vi "Global.vi"() -> ()   [LabVIEW 2020]
panel:
  in  "校验码":string
  in  "图号":string
  in  "法规号":string
  out "设备状态":i32
  in  "软件版本号":string
  in  "白/夜班":string
  in  "返工码":string
  in  "追溯代码":string
  in  "操作步骤":bool[](array[boolean])
  in  "更换型号":refnum<vi>
  in  "产品引用":refnum<vi>
  out "扭矩 2":sgl format="%#.3f"
  in  "扭矩":refnum<vi>
  out "传感器读数":T1 {"吸收电流" format="%#.3f"; "输出扭矩(大)" format="%#.3f"; "输出扭矩(小)" format="%#.3f"; "输入扭矩" format="%#.3f"; "输入编码位移" format="%#.3f"; "工装移载位移" format="%#.3f"; "输入移载位移" format="%#.3f"; "扭矩" format="%#.3f"}
  in  "CRC计数":u8
  in  "CAN_CYCLE":T2(array[cluster]) {"周期(ms)" min=1 format="%d ms"; "ID" format="0x%x"}
  in  "STOP_CAN":bool
  out "当前车速":u16
  in  "CAN Info":T3={"波特率"=11, "ID"=0, "帧类型"=enum."标准帧", "帧格式"=enum."数据帧", "周期(ms)"=10} {"周期(ms)" min=1 format="%d ms"; "ID" format="0x%x"; "波特率" items=["5Kbps", "10Kbps", "20Kbps", "40Kbps", "50Kbps", "80Kbps", "100Kbps", "125Kbps", "200Kbps", "250Kbps", "400Kbps", "500Kbps", "666Kbps", "800Kbps", "1000Kbps"]}
  in  "启用CAN":bool
  in  "合格数量 2":i32
  in  "生产数量 2":i32
  in  "计时开始":bool
  in  "计时复位":bool
  in  "前序状态":refnum<vi>
  in  "前序显示字":refnum<vi>
  in  "产品型号":string(combo)
  in  "结果显示":refnum<vi>
  in  "result":string
  in  "检测结果":refnum<vi>
  in  "合格数量":refnum<vi>
  in  "生产数量":refnum<vi>
  out "模式":u32
  in  "更换产品":refnum<vi>
  in  "提示信息":refnum<vi>
  in  "程序自动":refnum<vi>
  in  "报警图标":refnum<vi>
  in  "程序关闭":bool
  in  "Info":refnum<vi>
  in  "Result":refnum<vi>
  in  "批次":refnum<vi>
  # "帧ID"
  # "帧类型"
  # "帧格式"
  # "帧数据"
  # "周期"
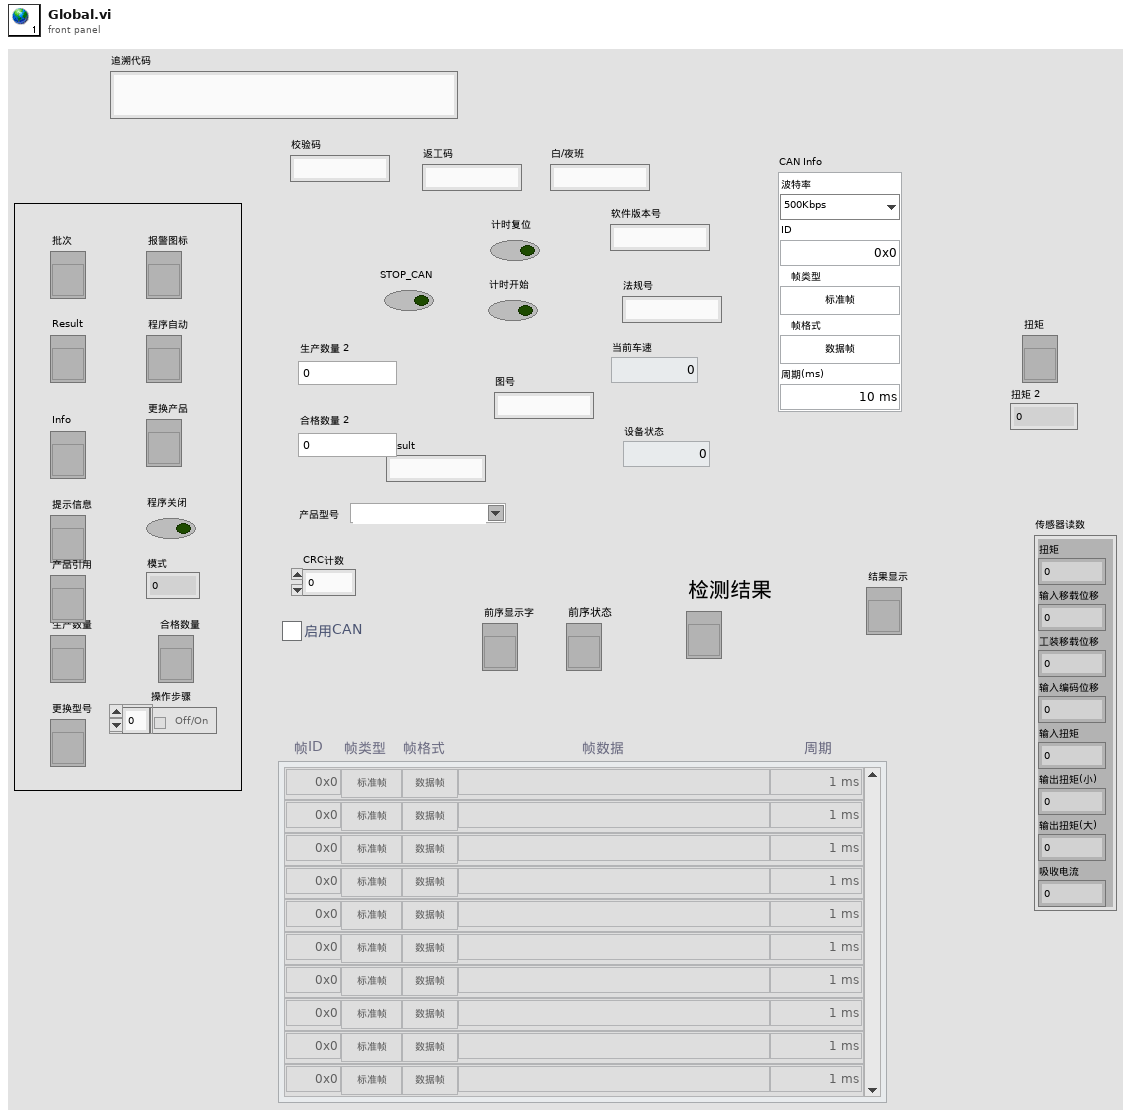
[diagram p1: front panel]
types:
  T1 = cluster{"扭矩":sgl, "输入移载位移":sgl, "工装移载位移":sgl, "输入编码位移":sgl, "输入扭矩":sgl, "输出扭矩(小)":sgl, "输出扭矩(大)":sgl, "吸收电流":sgl}
  T2 = cluster{"ID":u32, "帧类型":enum8{"标准帧", "扩展帧"}, "帧格式":enum16{"数据帧", "远程帧"}, "帧数据":string, "周期(ms)":u32}[]
  T3 = cluster{"波特率":u32, "ID":u32, "帧类型":enum8{"标准帧", "扩展帧"}, "帧格式":enum16{"数据帧", "远程帧"}, "周期(ms)":u32}
diagram:
